vi "LcWebView_AlertDialog_Custom with 3 buttons.vi"() -> ()   [LabVIEW 2018, in "LcWebView.lvclass"]
uses:
  LcWebView.lvclass
  C:/Projects/LcWebView2/LcWebView/LcWebView_class/data/Microsoft.Web.WebView2.WinForms.dll
  data/Microsoft.Web.WebView2.WinForms.dll
panel:
  out "BrowserProcessId":u32
  in  "stop":bool
  out "Status Message":string
  in  "Web":refnum<k24>(container)
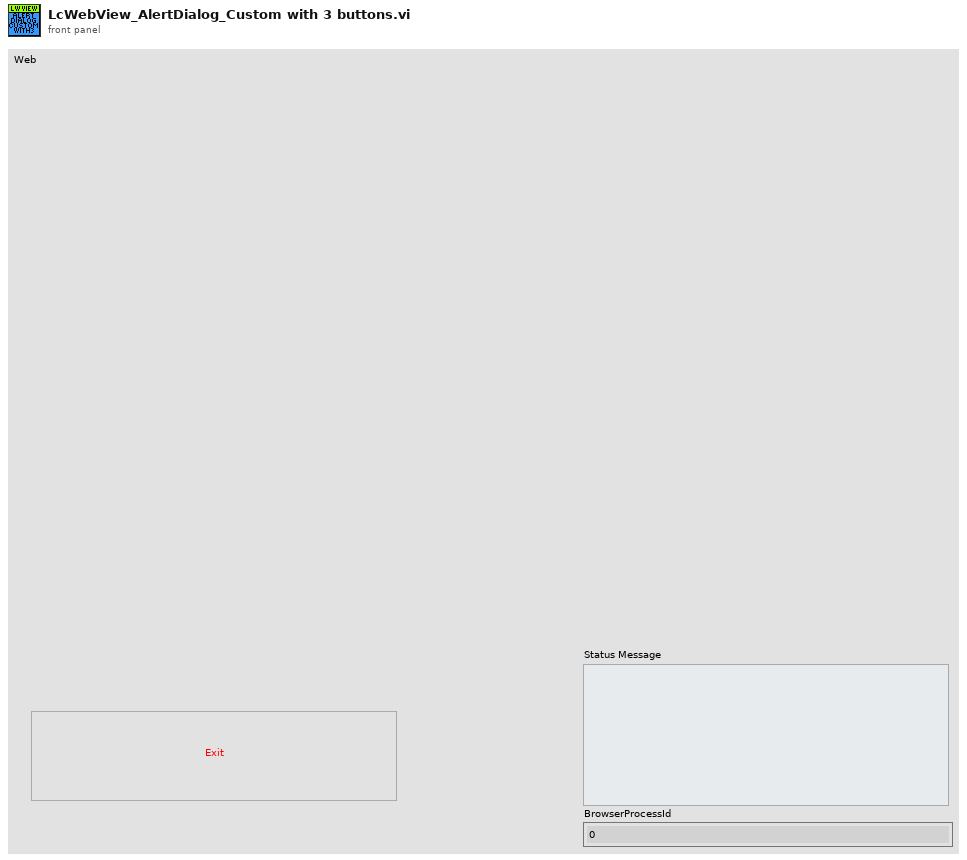
[diagram p1: front panel]
types:
  T1 = cluster{"title":string, "showDenyButton":bool, "showCancelButton":bool, "confirmButtonText":string, "denyButtonText":string}
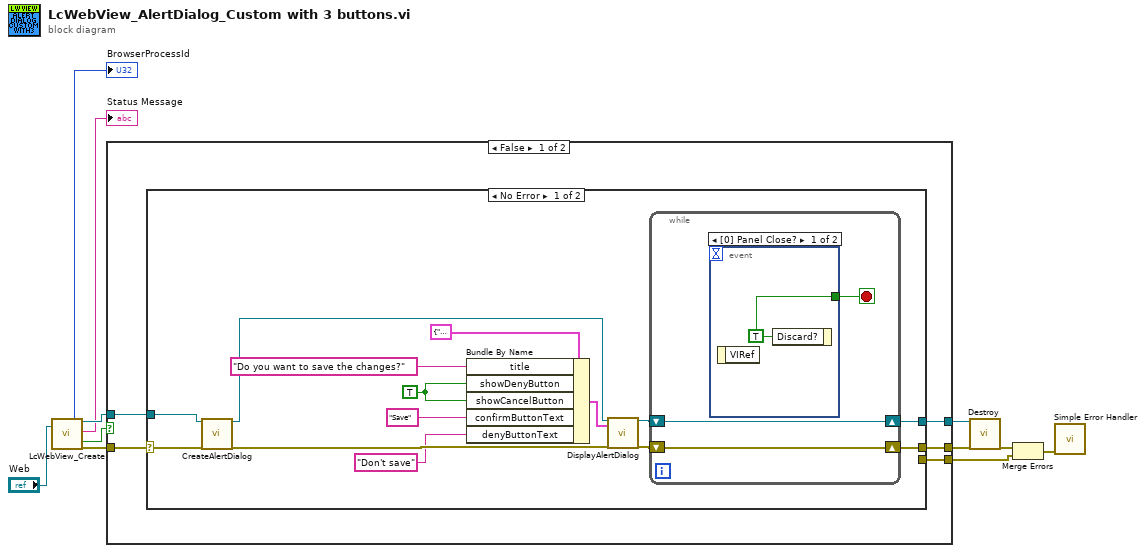
[diagram p0: block diagram]
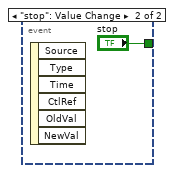
[diagram p2: hidden frame]
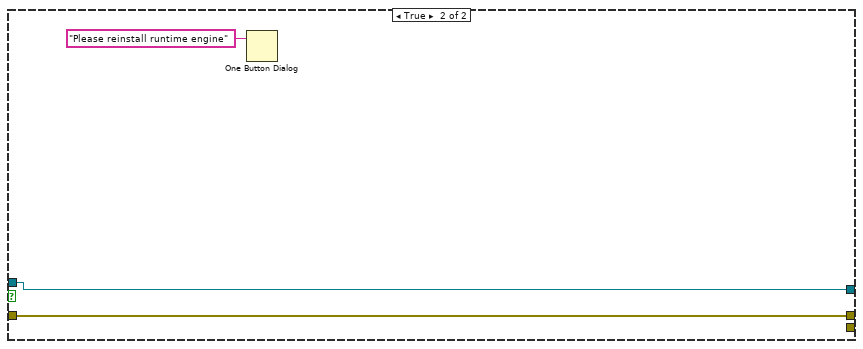
[diagram p4: hidden frame]
diagram:
  n1 = call "LcWebView_Create.vi"("Webview container"="Web") -> ("BrowserProcessId"=→"BrowserProcessId":u32, "reference out"=w10:refnum<class "LcWebView.lvclass">, "Status Message"=→"Status Message":string, "Reinstall Runtime"=w3:bool, "Error Out"=w9:errorcluster)  [unwired: 11 in, 3 out]
  n2 = case shown="False" w3 {
    tunnel: w10 -> [w16 w40]
    tunnel: w9 -> [w15 w39]
    tunnel: [w14 w40] -> w8
    tunnel: [w12 w39] -> w7
    tunnel: [w13 _] -> w4
    frame False {
      n3 = case shown="No Error" w15 {
        selector: w15 -> [w27 w36]
        tunnel: w16 -> [w28 w37]
        tunnel: [w29 w37] -> w14
        tunnel: [w30 _] -> w12
        tunnel: [_ w36] -> w13
        frame No Error {
          w19 = TRUE ("showDenyButton")
          n4 = call-dynamic "CreateAlertDialog.vi"("reference in"=w28, "Error In"=w27) -> ("reference out"=w26:refnum<class "LcWebView.lvclass">, "Error Out"=w25:errorcluster)  [unwired: 16 in]
          n5 = Bundle By Name(cluster=T1 {"title"="", "showDenyButton"=FALSE, "showCancelButton"=FALSE, "confirmButtonText"="", "denyButtonText"=""}, "title"="Do you want to save the changes?", "showDenyButton"=w19, "showCancelButton"=w19, "confirmButtonText"="Save", "denyButtonText"="Don't save") -> (w22:T1)
          n6 = call-dynamic "DisplayAlertDialog.vi"("reference in"=w26, "Message"=w22, "Error In"=w25) -> ("reference out"=w24:refnum<class "LcWebView.lvclass">, "Error Out"=w23:errorcluster)  [unwired: 14 in, 1 out]
          n7 = while {
            shift-right: [w33] -> w29
            shift-left: w24 -> [w33]
            shift-right: [w32] -> w30
            shift-left: w23 -> [w32]
            stop <- w31 stop-if-true
            n8 = event shown="[0] Panel Close?" {
              selector: _ -> [_ _]
              dyn-events: _ -> [_ _]
              timeout: _ -> [_ _]
              tunnel: [w34 "stop"] -> w31
              event Panel Close? {
                w34 = TRUE ("Discard?")
                n9 = event-data() -> ()  [unwired: 1 in, 1 out]
                n10 = event-data("Discard?"=w34) -> ()  [unwired: 1 in, 1 out]
              }
              event "stop": Value Change {
                n11 = event-data() -> ()  [unwired: 1 in, 6 out]
              }
            }
          }
        }
        frame Error {
        }
      }
    }
    frame True {
      n12 = One Button Dialog(message="Please reinstall runtime engine") -> ()  [unwired: 1 in, 1 out]
    }
  }
  n13 = call-dynamic "Destroy.vi"("reference in"=w8, "Error In"=w7) -> ("Error Out"=w6:errorcluster)  [unwired: 16 in, 1 out]
  n14 = Merge Errors(w6, w4) -> (w1:errorcluster)
  n15 = call <vilib>:"Simple Error Handler.vi"("error in (no error)"=w1) -> ()  [unwired: 4 in, 5 out]
